vi "TX_TakePhotoModule.vi"(8 "error out":errorcluster, 10 "Event Registration Refnum":refnum<event-registration>, 11 "queue out":refnum<queue>) -> (0 "error out 2":errorcluster)   [LabVIEW 2023]
uses:
  TX_Control 3.ctl
  <vilib>/vision/Image Controls.llb/IMAQ Image.ctl
  TX_Cluster1TypeDef.ctl
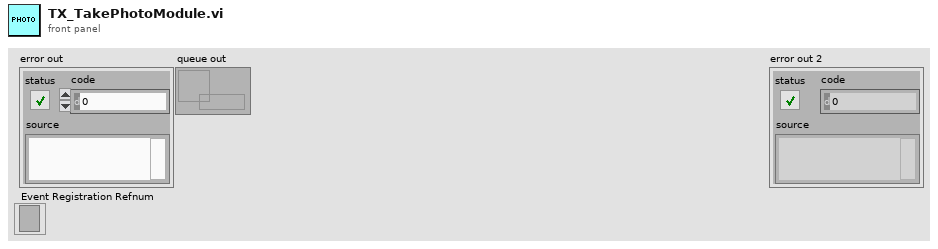
[diagram p1: front panel]
types:
  T1 = typedef "TX_Cluster1TypeDef.ctl" = cluster{"Enum":T2, "CamSel":variant, "CamView":variant}
  T2 = typedef "TX_Control 3.ctl" = enum16{"Default", "StartCamera", "TakePhoto", "EnableTCP", "Cam2Display", "CloseAll"}
  T3 = typedef "IMAQ Image.ctl" = refnum<image>
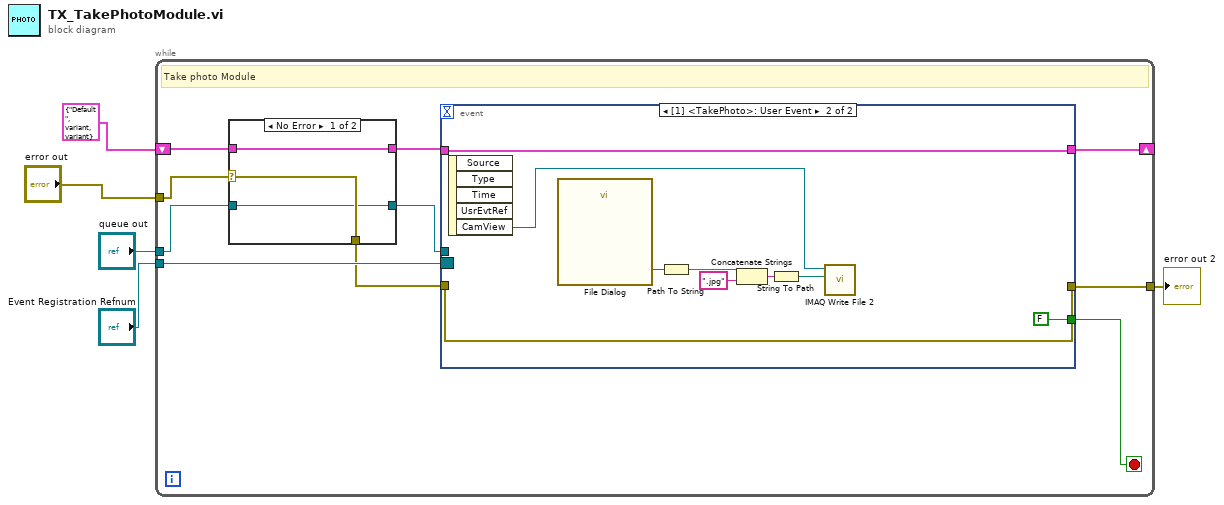
[diagram p0: block diagram]
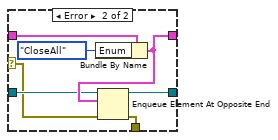
[diagram p2: hidden frame]
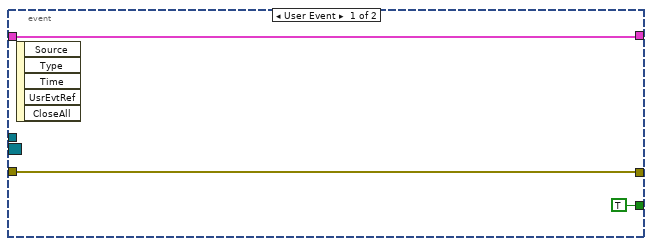
[diagram p3: hidden frame]
diagram:
  n1 = while {
    shift-right: [w13] -> _
    shift-left: T1 {"Enum"=enum."Default", "CamSel"=variant(refnum<image> refnum), "CamView"=variant(refnum<image> refnum)} ("Cluster") -> [w10]
    tunnel: "Event Registration Refnum" -> [w15]
    tunnel: "queue out" -> [w7]
    tunnel: "error out" -> [w11]
    tunnel: [w14] -> w1
    stop <- w12 stop-if-true
    # "Take photo Module"
    n2 = case shown="No Error" w11 {
      selector: w11 -> [w17 w21]
      tunnel: [w18 w23] -> w9
      tunnel: w10 -> [w18 w25]
      tunnel: w7 -> [w16 w22]
      tunnel: [w17 w20] -> w8
      tunnel: [w16 w19] -> w6
      frame No Error {
      }
      frame Error {
        n3 = Bundle By Name(cluster=w25, "Enum"=TX_Control_3."CloseAll") -> (w23:T1)
        n4 = Enqueue Element At Opposite End(queue=w22, element=w23, error in (no error)=w21) -> (queue out=w19:refnum<queue>, error out=w20:errorcluster)  [unwired: 1 in, 1 out]
      }
    }
    n5 = event shown="[1] <TakePhoto>: User Event" {
      selector: w15 -> [_ _]
      dyn-events: _ -> [_ _]
      timeout: _ -> [_ _]
      tunnel: [w27 w35] -> w13
      tunnel: w9 -> [w27 w35]
      tunnel: w6 -> [_ _]
      tunnel: w8 -> [w26 w36]
      tunnel: [w26 w36] -> w14
      tunnel: [TRUE FALSE] -> w12
      event User Event {
        n6 = event-data() -> ()  [unwired: 1 in, 5 out]
      }
      event User Event {
        n7 = event-data() -> ("CamView"=w29:T3)  [unwired: 1 in, 4 out]
        n8 = call "File Dialog"() -> ("selected path"=w34:path)  [unwired: 12 in, 3 out]
        n9 = Path To String(path=w34) -> (string=w33:string)
        n10 = Concatenate Strings(w33, ".jpg" ("string")) -> (w31:string)
        n11 = String To Path(string=w31) -> (path=w30:path)
        n12 = call-poly "IMAQ Write File 2"("File Path"=w30, "Image"=w29) -> ()  [unwired: 8 in, 2 out]
      }
    }
  }
  "error out 2" <- w1
